vi "voltage up voltage down1.vi"() -> ()   [LabVIEW 2017]
panel:
  in  "stop":bool
  in  "operation (0:open)":T1(ring)
  in  "file path (use dialog)":path
  in  "Vstep":dbl
  in  "Vmin":dbl
  in  "Vmax":dbl
  in  "wait time":dbl
  out "Current vs Voltage":cluster{dbl[], dbl[]}(graph)
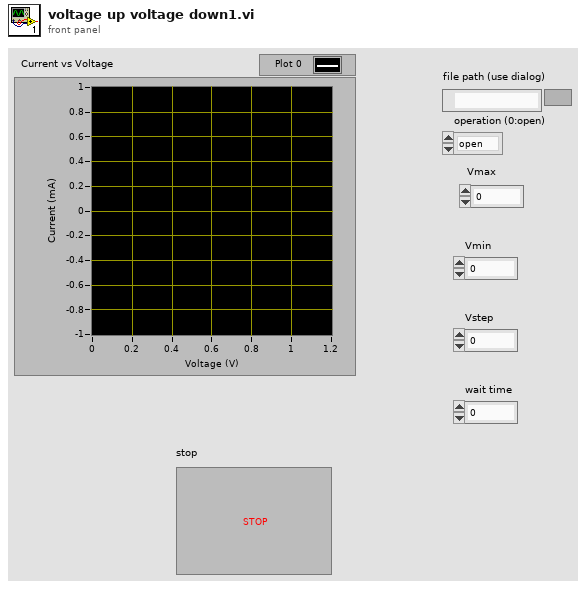
[diagram p1: front panel]
types:
  T1 = enum16{"open", "replace", "create", "open or create", "replace or create", "replace or create with confirmation"}
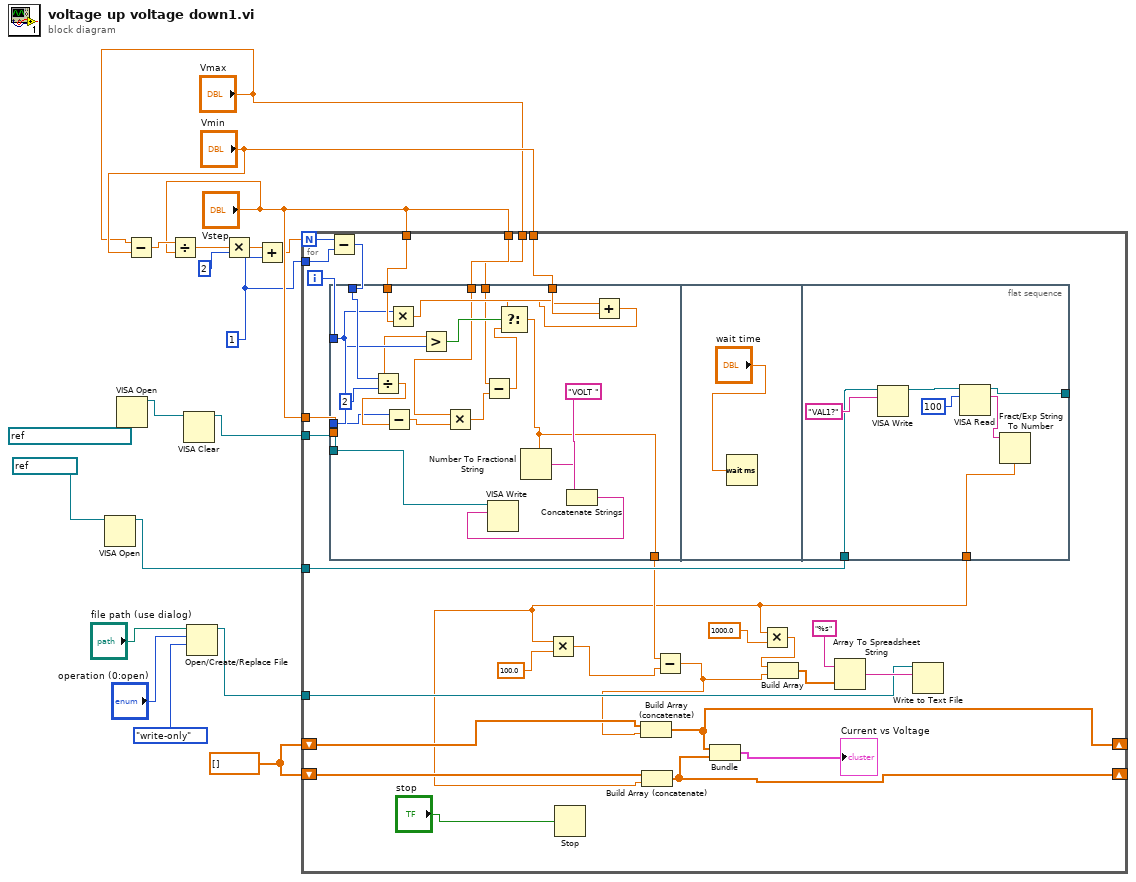
[diagram p0: block diagram]
diagram:
  w1 = dbl[] []
  w9 = 1
  n1 = VISA Open(VISA resource name=refnum<visa-resource-name> "Fluke45" ("Fluke")) -> (VISA resource name=w6:refnum<visa-resource-name>)  [unwired: 4 in, 1 out]
  n2 = VISA Open(VISA resource name=refnum<visa-resource-name> "AgilentPowerSupply" ("AgilentPower")) -> (VISA resource name=w15:refnum<visa-resource-name>)  [unwired: 4 in, 1 out]
  n3 = Subtract(x="Vmax", y="Vmin") -> (x-y=w19:dbl)
  n4 = Divide(x=w19, y="Vstep") -> (x/y=w17:dbl)
  n5 = VISA Clear(VISA resource name=w15) -> (VISA resource name out=w14:refnum<visa-resource-name>)  [unwired: 1 in, 1 out]
  n6 = Open/Create/Replace File(file path (use dialog)="file path (use dialog)", operation (0:open)="operation (0:open)", access (0:read/write)=enum16{"read/write", "read-only", "write-only"}."write-only") -> (refnum out=w4:refnum<file>)  [unwired: 3 in, 2 out]
  n7 = Multiply(x=w17, y=2) -> (x*y=w11:dbl)
  n8 = Add(x=w11, y=w9) -> (x+y=w10:dbl)
  n9 = for {
    N: w10 -> [w41]
    tunnel: "Vstep" -> [w47]
    tunnel: w14 -> [w46]
    tunnel: "Vmin" -> [w45]
    tunnel: "Vstep" -> [w44]
    tunnel: "Vstep" -> [w43]
    tunnel: w9 -> [w40]
    tunnel: "Vmax" -> [w38]
    tunnel: w6 -> [w37]
    tunnel: w4 -> [w28]
    shift-right: [w22] -> _
    shift-left: w1 -> [w27]
    shift-right: [w21] -> _
    shift-left: w1 -> [w26]
    i -> [w42]
    n10 = Subtract(x=w41, y=w40) -> (x-y=w39:i32)
    n11 = flat-sequence {
      tunnel: w39 -> [w61]
      tunnel: w47 -> [_]
      tunnel: w46 -> [w65]
      tunnel: w45 -> [w64]
      tunnel: w42 -> [w60]
      tunnel: w44 -> [w63]
      tunnel: w43 -> [w59]
      tunnel: w42 -> [w50]
      tunnel: w38 -> [w49]
      tunnel: [w48] -> w34
      tunnel: w37 -> [w72]
      tunnel: [w71] -> _
      tunnel: [w69] -> w24
      frame #0 {
        n12 = Divide(x=w61, y=2) -> (x/y=w51:dbl)
        n13 = Subtract(x=w50, y=w51) -> (x-y=w52:dbl)
        n14 = Multiply(x=w60, y=w63) -> (x*y=w62:dbl)
        n15 = Greater?(x=w51, y=w60) -> (0:w66:bool)
        n16 = Multiply(x=w59, y=w52) -> (x*y=w58:dbl)
        n17 = Subtract(x=w49, y=w58) -> (x-y=w57:dbl)
        n18 = Add(x=w62, y=w64) -> (x+y=w56:dbl)
        n19 = Select(t=w56, s=w66, f=w57) -> (s? t:f=w48:dbl)
        n20 = Number To Fractional String(number=w48) -> (F-format string=w54:string)  [unwired: 3 in]
        n21 = Concatenate Strings("VOLT ", w54) -> (w53:string)
        n22 = VISA Write(VISA resource name=w65, write buffer=w53) -> ()  [unwired: 1 in, 3 out]
      }
      frame #1 {
        n23 = Wait (ms)(milliseconds to wait="wait time") -> ()  [unwired: 1 out]
      }
      frame #2 {
        n24 = VISA Write(VISA resource name=w72, write buffer="VAL1?") -> (VISA resource name out=w75:refnum<visa-resource-name>)  [unwired: 1 in, 2 out]
        n25 = VISA Read(VISA resource name=w75, byte count=100) -> (VISA resource name out=w71:refnum<visa-resource-name>, read buffer=w70:string)  [unwired: 1 in, 2 out]
        n26 = Fract/Exp String To Number(string=w70) -> (number=w69:dbl)  [unwired: 3 in, 1 out]
      }
    }
    n27 = Multiply(x=w24, y=100.0) -> (x*y=w35:dbl)
    n28 = Stop(stop? (T)="stop") -> ()
    n29 = Build Array (concatenate)(w26, w24) -> (w21:dbl[])
    n30 = Subtract(x=w34, y=w35) -> (x-y=w25:dbl)
    n31 = Build Array (concatenate)(w27, w25) -> (w22:dbl[])
    n32 = Bundle(w22, w21) -> (→"Current vs Voltage":cluster{dbl[], dbl[]})  [unwired: 1 in]
    n33 = Multiply(x=w24, y=1000.0) -> (x*y=w33:dbl)
    n34 = Build Array(w33, w25) -> (w31:dbl[])
    n35 = Array To Spreadsheet String(array=w31, 3:"%s") -> (spreadsheet string=w29:string)  [unwired: 1 in]
    n36 = Write to Text File(file (use dialog)=w28, text=w29) -> ()  [unwired: 2 in, 3 out]
  }
